vi "SectionName-VacuumLine.vi"(1 "VacuumLine Configuration in":refnum<class "VacuumLine Configuration.lvclass">) -> (0 "SectionName":string)   [LabVIEW 2016, in "Hardware.lvlib" / "VacuumLine.lvlib" / "VacuumLine Configuration.lvclass"]
uses:
  <userlib>/Common Components/Hardware/Abstract System/VacuumLine/VacuumLine Config/VacuumLine Configuration.lvclass
  <userlib>/Common Components/Hardware/Abstract System/VacuumLine/VacuumLine Config/VacuumLine Configuration.lvclass/VacuumLine Configuration.ctl
  <userlib>/Common Components/Hardware/Abstract System/VacuumLine/VacuumLine/VacuumLine.lvclass/VacuumLine.ctl
  <userlib>/Common Components/Hardware/Abstract System/VacuumLine/VacuumLine/Read Label.vi
  <userlib>/Common Components/Hardware/Abstract System/VacuumLine/VacuumLine/VacuumLine.lvclass
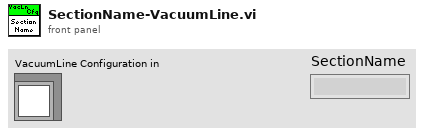
[diagram p1: front panel]
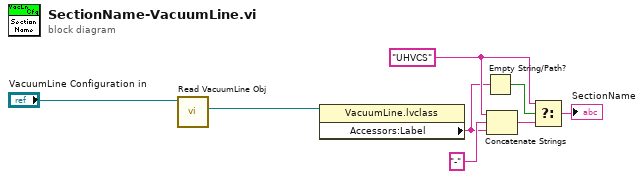
[diagram p0: block diagram]
diagram:
  w5 = "UHVCS"
  n1 = call <userlib>:"Read VacuumLine Obj.vi"("VacuumLine Configuration in"="VacuumLine Configuration in") -> ("Hardware.lvlib:VacuumLine.lvlib:VacuumLine.lvclass"=w7:refnum<class "VacuumLine.lvclass">)  [unwired: 8 in, 2 out]
  n2 = property class="VacuumLine.lvclass"(reference=w7) -> ("Accessors:Label"=w3:string)  [unwired: 1 in, 2 out]
  n3 = Empty String/Path?(string/path=w3) -> (empty?=w6:bool)
  n4 = Concatenate Strings(w5, "-" ("string"), w3) -> (w2:string)
  n5 = Select(t=w5, s=w6, f=w2) -> (s? t:f=→"SectionName":string)
